vi "Git-Get Commits from Repository API-URL.vi"(8 "error in (no error)":errorcluster, 11 "Repository API URL":string) -> (0 "error out":errorcluster, 3 "Commits":T1[](array[typedef]))   [LabVIEW 2020]
uses:
  Git-Committ JSON Typedef.ctl
  <vilib>/JDP Science/JSONtext/String Subset.vi
  <vilib>/JDP Science/JSONtext/Parsing/Parse Full Path or Item Name.vi
  <vilib>/JDP Science/JSONtext/Offset/Find Item Locations by Path.vi
  <vilib>/addons/_JKI.lib/REST Client/classes/REST Client/REST Client.lvclass
  <vilib>/JDP Science/JSONtext/JSONtext.lvlib
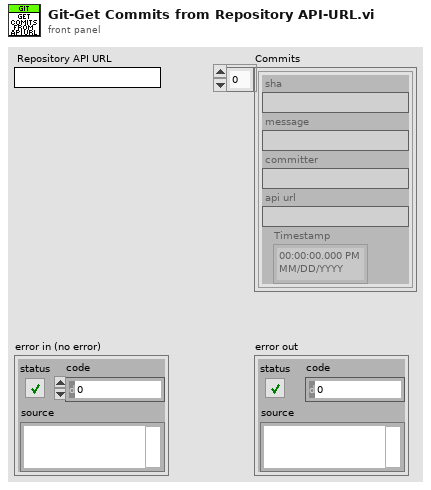
[diagram p1: front panel]
types:
  T1 = typedef "Git-Committ JSON Typedef.ctl" = cluster{"sha":string, "message":string, "committer":string, "api url":string, "Timestamp":timestamp}
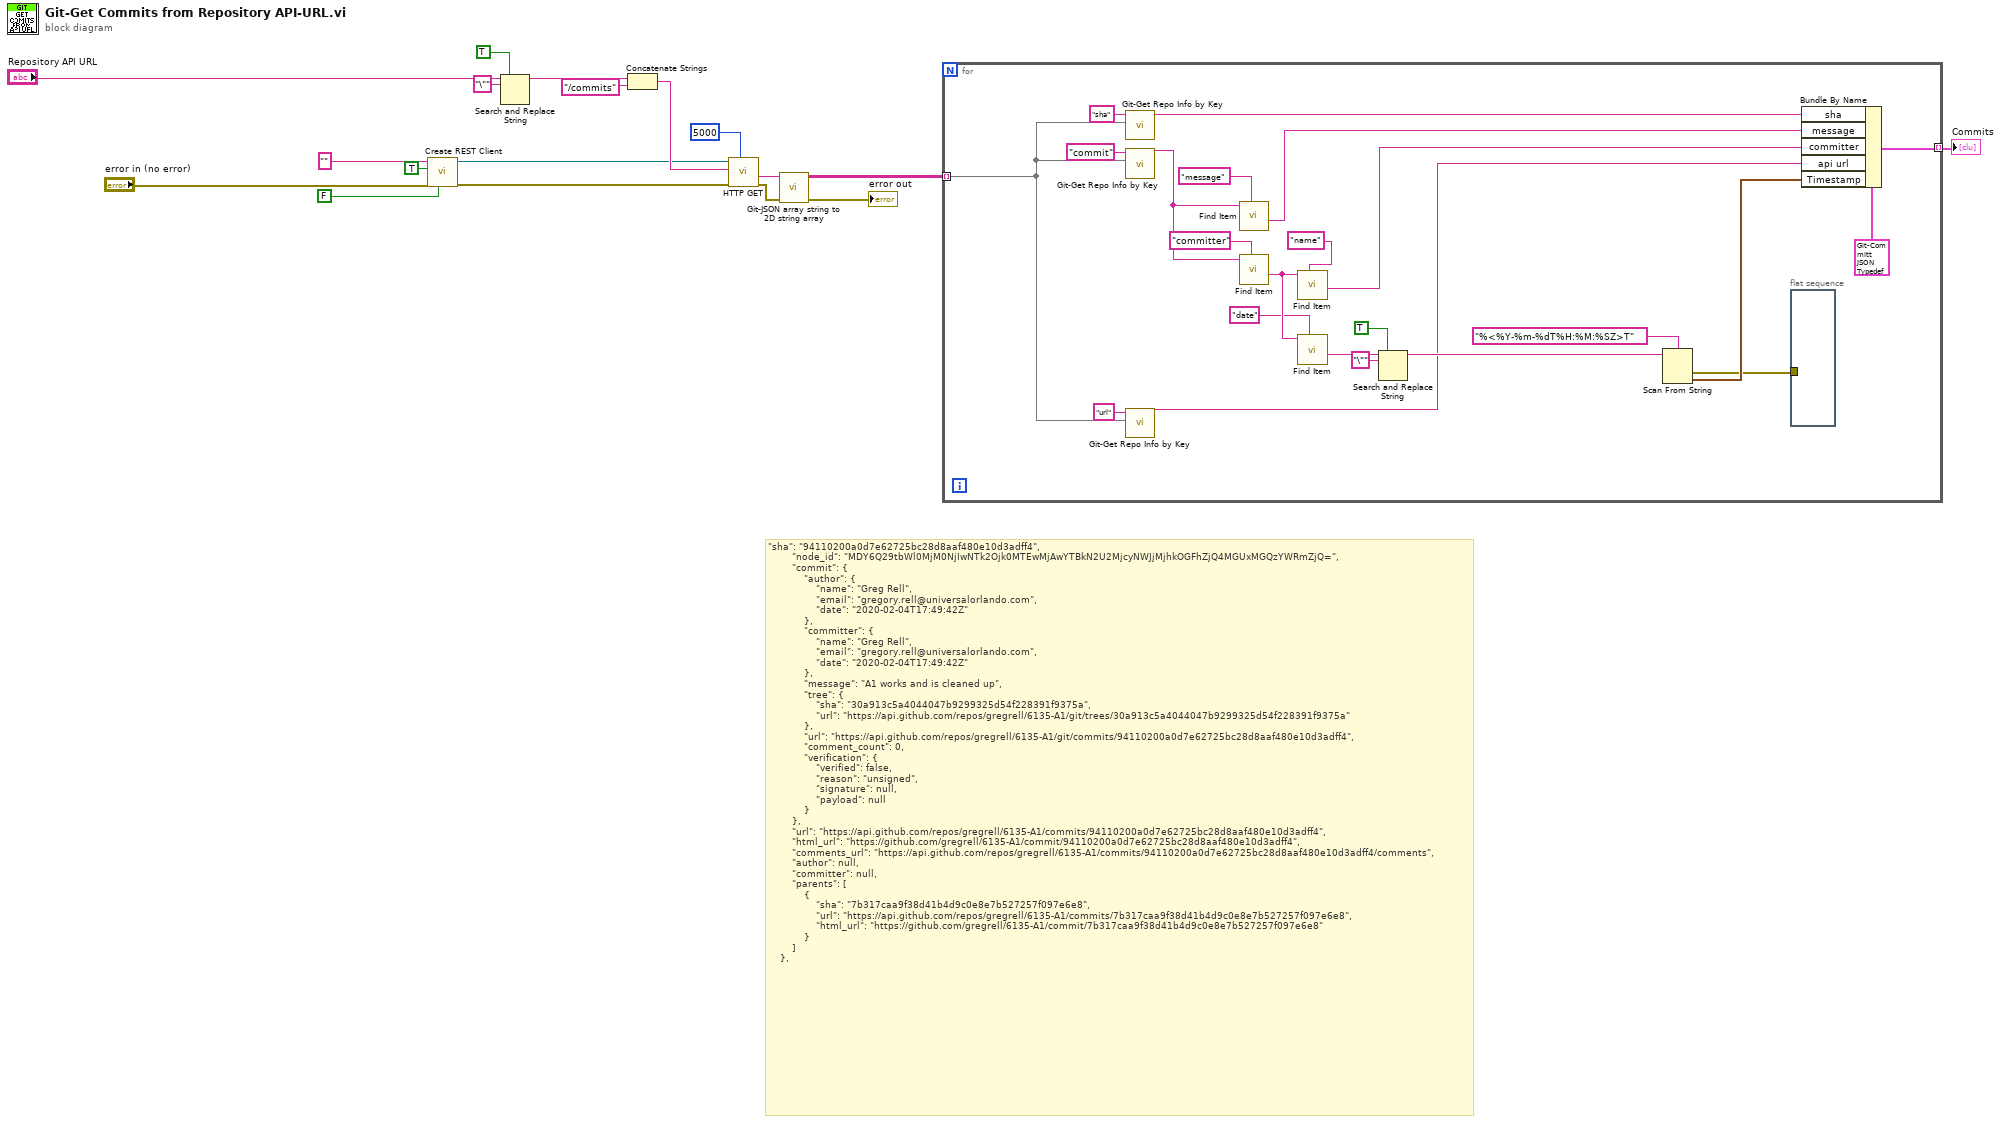
[diagram p0: block diagram]
diagram:
  # "\"sha\": \"94110200a0d7e62725bc28d8aaf480e10d3adff4\",\n        \"node_id\": \"MDY6Q29tbWl0MjM0NjIwNTk2Ojk0MTEwMjAwYTBkN2U2MjcyNWJjMjhkOGFhZjQ4MGUxMGQzYWRmZjQ=\",\n        \"commit\": {\n            \"author\": {\n                \"name\": \"Greg Rell\",\n                \"email\": \"gregory.rell@universalorlando.com\",\n                \"date\": \"2020-02-04T17:49:42Z\"\n            },\n            \"committer\": {\n                \"name\": \"Greg Rell\",\n                \"email\": \"gregory.rell@universalorlando.com\",\n                \"date\": \"2020-02-04T17:49:42Z\"\n            },\n            \"message\": \"A1 works and is cleaned up\",\n            \"tree\": {\n                \"sha\": \"30a913c5a4044047b9299325d54f228391f9375a\",\n                \"url\": \"https://api.github.com/repos/gregrell/6135-A1/git/trees/30a913c5a4044047b9299325d54f228391f9375a\"\n            },\n            \"url\": \"https://api.github.com/repos/gregrell/6135-A1/git/commits/94110200a0d7e62725bc28d8aaf480e10d3adff4\",\n            \"comment_count\": 0,\n            \"verification\": {\n                \"verified\": false,\n                \"reason\": \"unsigned\",\n                \"signature\": null,\n                \"payload\": null\n            }\n        },\n        \"url\": \"https://api.github.com/repos/gregrell/6135-A1/commits/94110200a0d7e62725bc28d8aaf480e10d3adff4\",\n        \"html_url\": \"https://github.com/gregrell/6135-A1/commit/94110200a0d7e62725bc28d8aaf480e10d3adff4\",\n        \"comments_url\": \"https://api.github.com/repos/gregrell/6135-A1/commits/94110200a0d7e62725bc28d8aaf480e10d3adff4/comments\",\n        \"author\": null,\n        \"committer\": null,\n        \"parents\": [\n            {\n                \"sha\": \"7b317caa9f38d41b4d9c0e8e7b527257f097e6e8\",\n                \"url\": \"https://api.github.com/repos/gregrell/6135-A1/commits/7b317caa9f38d41b4d9c0e8e7b527257f097e6e8\",\n                \"html_url\": \"https://github.com/gregrell/6135-A1/commit/7b317caa9f38d41b4d9c0e8e7b527257f097e6e8\"\n            }\n        ]\n    },"
  n1 = call <vilib>:"Create REST Client.vi"("Verify Server(true)"=FALSE, "error in (no error)"="error in (no error)", "Escape URLs (true)"=TRUE, "Base URL"="") -> ("error out"=w3:errorcluster, "REST Client out"=w5:refnum<class "REST Client.lvclass">)  [unwired: 6 in]
  n2 = Search and Replace String(replace all?=TRUE ("replace all? (F)"), input string="Repository API URL", search string="\"") -> (result string=w12:string)  [unwired: 5 in, 3 out]
  n3 = Concatenate Strings(w12, "/commits" ("string")) -> (w13:string)
  n4 = call-dynamic "HTTP GET.vi"("timeout (0 = Use Default)"=5000, "error in (no error)"=w3, "Path"=w13, "REST Client in"=w5) -> ("error out"=w16:errorcluster, "Response body"=w14:string)  [unwired: 2 in, 4 out]
  n5 = call "Git-JSON array string to 2D string array.vi"("error in (no error)"=w16, "Response body"=w14) -> ("error out"=→"error out":errorcluster, "Array"=w15:string[][][])  [unwired: 8 in]
  n6 = for {
    tunnel: w15 -> [w21] mode=indexing
    tunnel: [w39] -> w18 mode=indexing
    n7 = call "Git-Get Repo Info by Key.vi"("Repo Info"=w21, "Key"="sha" ("element")) -> ("<JSON>"=w40:string)  [unwired: 9 in]
    n8 = call "Git-Get Repo Info by Key.vi"("Repo Info"=w21, "Key"="commit" ("element")) -> ("<JSON>"=w33:string)  [unwired: 9 in]
    n9 = call "Git-Get Repo Info by Key.vi"("Repo Info"=w21, "Key"="url" ("element")) -> ("<JSON>"=w20:string)  [unwired: 9 in]
    n10 = call <vilib>:"Find Item.vi"("$Path or Item Name"="message", "JSON"=w33) -> ("<JSON>"=w35:string)  [unwired: 6 in, 3 out]
    n11 = call <vilib>:"Find Item.vi"("$Path or Item Name"="committer", "JSON"=w33) -> ("<JSON>"=w30:string)  [unwired: 6 in, 3 out]
    n12 = call <vilib>:"Find Item.vi"("$Path or Item Name"="name", "JSON"=w30) -> ("<JSON>"=w31:string)  [unwired: 6 in, 3 out]
    n13 = call <vilib>:"Find Item.vi"("$Path or Item Name"="date", "JSON"=w30) -> ("<JSON>"=w28:string)  [unwired: 6 in, 3 out]
    n14 = Search and Replace String(replace all?=TRUE ("replace all? (F)"), input string=w28, search string="\"") -> (result string=w24:string)  [unwired: 5 in, 3 out]
    n15 = Scan From String(format string="%<%Y-%m-%dT%H:%M:%SZ>T", input string=w24) -> (error out=w19:errorcluster, output 1=w23:timestamp)  [unwired: 3 in, 2 out]
    n16 = flat-sequence {
      tunnel: w19 -> [_]
      frame #0 {
      }
    }
    n17 = Bundle By Name(cluster=T1 {"sha"="", "message"="", "committer"="", "api url"="", "Timestamp"=timestamp(0 s since 1904-01-01)}, "sha"=w40, "message"=w35, "committer"=w31, "api url"=w20, "Timestamp"=w23) -> (w39:T1)
  }
  "Commits" <- w18
